vi "practice04_voltage_serial.vi"() -> ()   [LabVIEW 2025]
uses:
  <vilib>/Instr/_visa.llb/VISA Configure Serial Port (Instr).vi
panel:
  out "Voltaje":string
  in  "Muestreo":u32
  in  "stop":bool
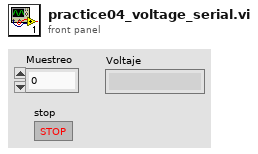
[diagram p1: front panel]
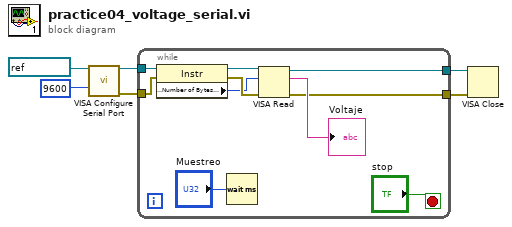
[diagram p0: block diagram]
diagram:
  n1 = call-poly "VISA Configure Serial Port"("VISA resource name"=refnum<visa-resource-name> "COM3", "parity (0:none)"=9600) -> ("VISA resource name out"=w2:refnum<visa-resource-name>, "error out"=w1:errorcluster)  [unwired: 12 in]
  n2 = while {
    tunnel: [w11] -> w6
    tunnel: [w10] -> w5
    tunnel: w2 -> [w8]
    tunnel: w1 -> [w7]
    stop <- "stop" stop-if-true
    n3 = property class="Instr"(reference=w8, error in=w7) -> (reference out=w9:refnum<visa-resource-name>, error out=w14:errorcluster, "Serial Settings:Number of Bytes at Serial Port"=w13:u32)
    n4 = Wait (ms)(milliseconds to wait="Muestreo") -> ()  [unwired: 1 out]
    n5 = VISA Read(VISA resource name=w9, byte count=w13, error in (no error)=w14) -> (VISA resource name out=w11:refnum<visa-resource-name>, read buffer=→"Voltaje":string, error out=w10:errorcluster)  [unwired: 1 out]
  }
  n6 = VISA Close(VISA resource name=w6, error in (no error)=w5) -> ()  [unwired: 1 out]
